vi "MVP02_P_CD.vi"() -> ()   [LabVIEW 2016]
uses:
  <vilib>/xnet/xnet.llb/XNET Read (Signal Waveform) .vi
  <vilib>/Waveform/WDTOps.llb/WDT Append Waveforms DBL.vi
  <vilib>/Waveform/WDTOps.llb/WDT Number of Waveform Samples DBL.vi
  <vilib>/measure/matone.llb/Extract Single Tone Information 1 Chan.vi
  <vilib>/measure/mamon.llb/Create Continuous Mask.vi
  <vilib>/measure/mamon.llb/Limit Testing Time.vi
  Custom Device/MVP02/MVP02 Custom Device.lvlib
  <vilib>/measure/NI_MAPro.lvlib
  <vilib>/measure/NI_MABase.lvlib
panel:
  out "error out 6":errorcluster
  out "Waveform Graph":waveform(dbl)[](graph)
  out "test passed?":bool
  out "error out 4":errorcluster
  out "error out 3":errorcluster caption="error out"
  out "error out 2":errorcluster caption="error out"
  in  "signal type":T1(ring)
  in  "error in (no error)":errorcluster
  out "error out":errorcluster
  in  "Repeticao":dbl format="%#_13g"
  in  "Caso Teste":dbl format="%#_13g"
  out "Gabarito":string
  out "String (OCR/OCV 1)":string
  out "Passed?":bool
  in  "milliseconds to wait":u32=100
  in  "stop":bool
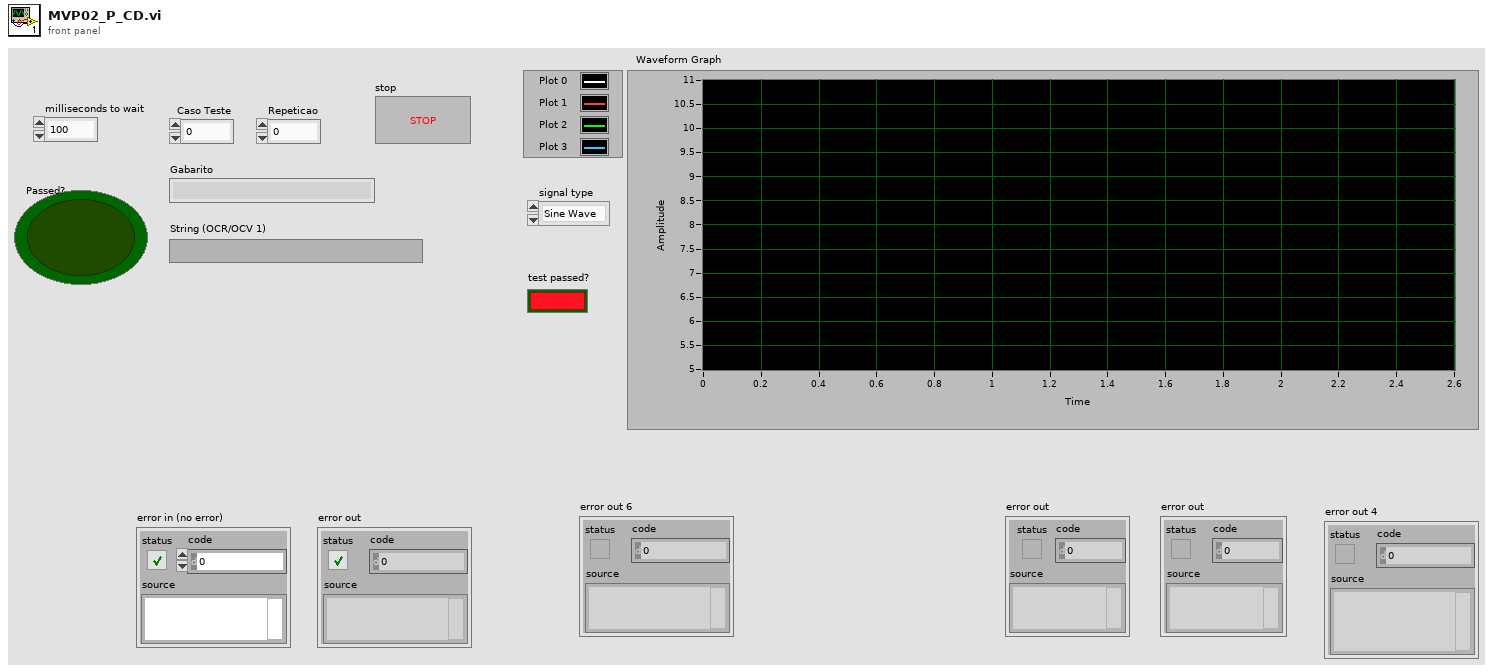
[diagram p1: front panel]
types:
  T1 = enum16{"Sine Wave", "Triangle Wave", "Square Wave", "Sawtooth Wave"}
  T2 = cluster{"pass region":i32, "include UL":bool, "include LL":bool}
  T3 = typedef "Vision Case.ctl" = enum16{"Espera", "OCR", "OCR2", "Outros"}
  T4 = typedef "IMAQ Image.ctl" = refnum<image>
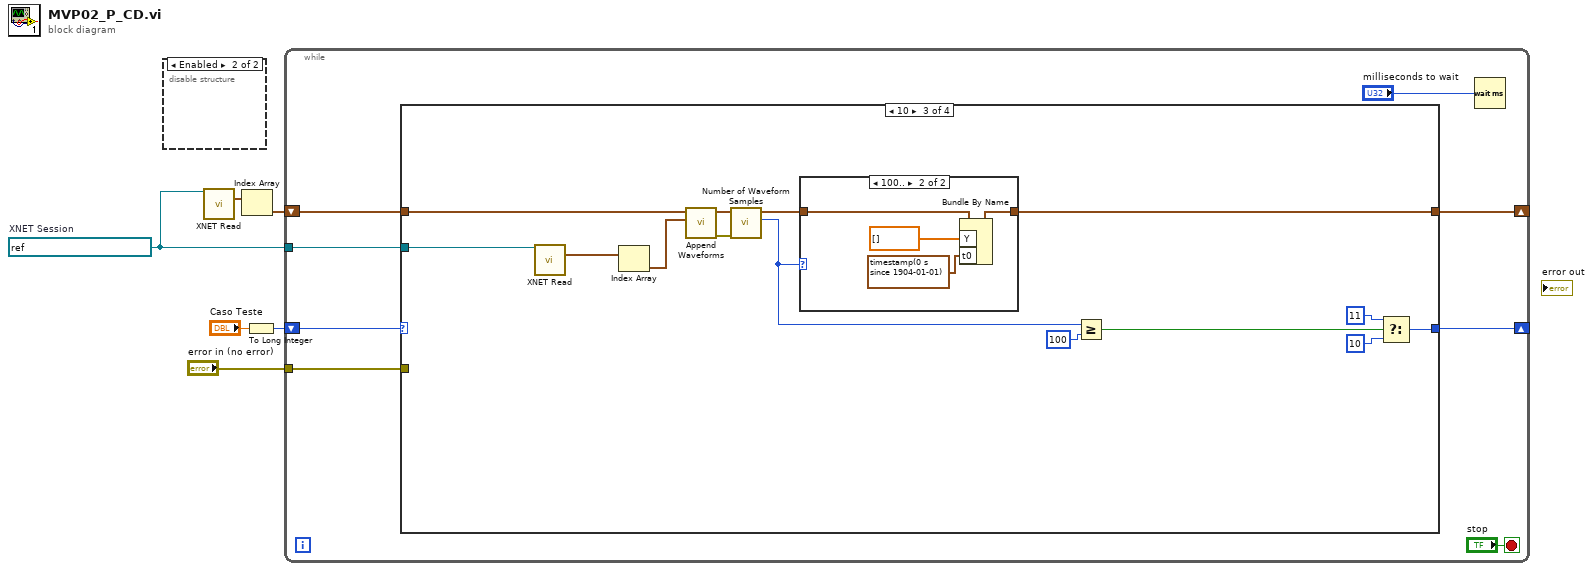
[diagram p0: block diagram]
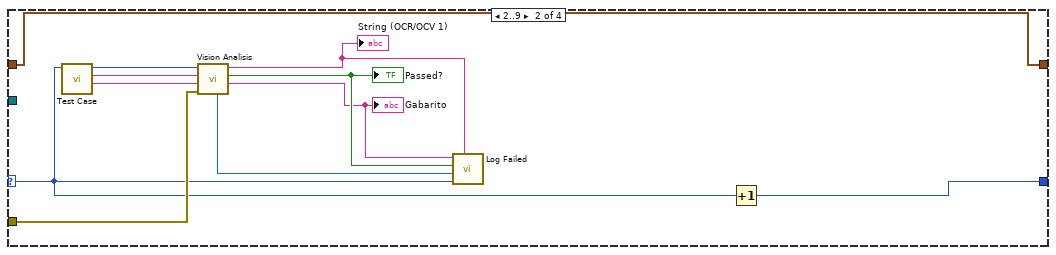
[diagram p3: hidden frame]
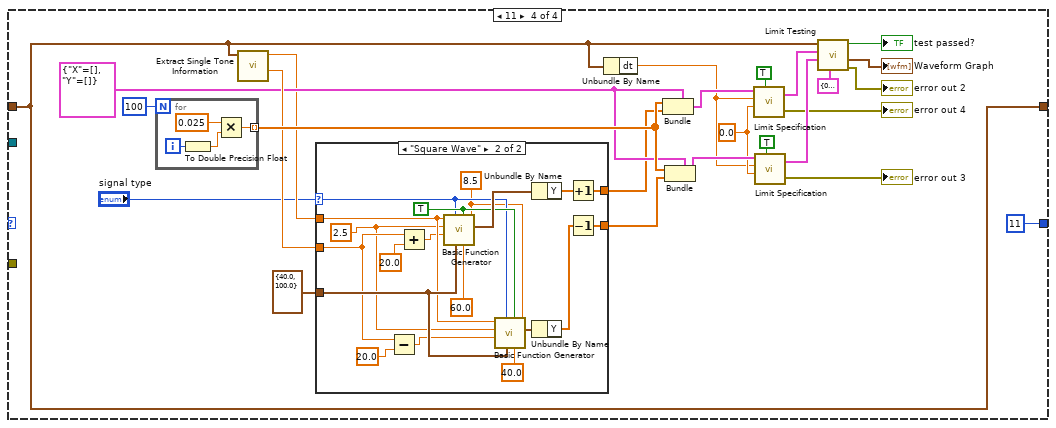
[diagram p5: hidden frame]
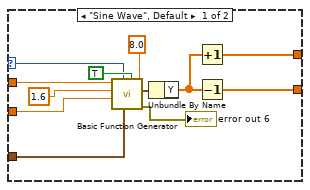
[diagram p6: hidden frame]
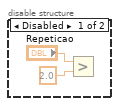
[diagram p7: hidden frame]
diagram:
  w2 = refnum<k21> "New NI-XNET Session"  # XNET Session
  n1 = disable-structure shown="Enabled" {
    frame Disabled {
      n2 = Greater?(x="Repeticao", y=2.0) -> ()  [unwired: 1 out]
    }
    frame Enabled {
    }
  }
  n3 = call-poly <vilib>:"XNET Read.vi"("session in"=w2) -> ("data"=w3:waveform(dbl)[])  [unwired: 12 in, 2 out]
  n4 = Index Array(array=w3) -> (element=w1:waveform(dbl))  [unwired: 1 in]
  n5 = To Long Integer(number="Caso Teste") -> (32bit integer=w4:i32)
  n6 = while {
    tunnel: "error in (no error)" -> [w14]
    shift-right: [w13] -> _
    shift-left: w4 -> [w12]
    tunnel: w2 -> [w11]
    shift-right: [w9] -> _
    shift-left: w1 -> [w10]
    stop <- "stop" stop-if-true
    n7 = case shown="10" w12 {
      selector: w12 -> [w18 w21 _ _]
      tunnel: w14 -> [_ w29 _ _]
      tunnel: [w18 w20 w34 11 ("32bit integer")] -> w13
      tunnel: w11 -> [_ _ w42 _]
      tunnel: w10 -> [w17 w19 w41 w50]
      tunnel: [w17 w19 w35 w50] -> w9
      frame 0, Default {
      }
      frame 2..9 {
        n8 = call "Test Case.vi"("Numeric"=w21) -> ("Linha 2"=w26:string, "Linha 1"=w27:string, "Image Case"=w28:T3)  [unwired: 8 in]
        n9 = call "Vision Analisis.vi"("error in"=w29, "Linha 2"=w26, "Linha 1"=w27, "Image Case"=w28) -> ("Gabarito"=w23:string, "Passed?"=w24:bool, "String (OCR/OCV 1)"=w22:string, "Image Out"=w25:T4)  [unwired: 3 in, 1 out]
        "Passed?" <- w24
        "String (OCR/OCV 1)" <- w22
        "Gabarito" <- w23
        n10 = call "Log Failed.vi"("RESULTADO"=w22, "Case number"=w21, "Image In"=w25, "Boolean"=w24, "GABARITO"=w23) -> ()  [unwired: 7 in]
        n11 = Increment(x=w21) -> (x+1=w20:i32)
      }
      frame 10 {
        n12 = call-poly <vilib>:"XNET Read.vi"("session in"=w42) -> ("data"=w40:waveform(dbl)[])  [unwired: 12 in, 2 out]
        n13 = Index Array(array=w40) -> (element=w39:waveform(dbl))  [unwired: 1 in]
        n14 = call-poly <vilib>:"Append Waveforms.vi"("waveform B"=w39, "waveform A"=w41) -> ("error out"=w38:errorcluster, "waveform out"=w37:waveform(dbl))  [unwired: 8 in]
        n15 = call-poly <vilib>:"Number of Waveform Samples.vi"("error in (no error)"=w38, "waveform in"=w37) -> ("number of samples"=w31:i32, "waveform out"=w36:waveform(dbl))  [unwired: 7 in, 1 out]
        n16 = case shown="100.." w31 {
          tunnel: w36 -> [w44 w45]
          tunnel: [w44 w48] -> w35
          frame 0, Default {
          }
          frame 100.. {
            n17 = Bundle By Name(cluster=w45, "Y"=dbl[] [], "t0"=timestamp(0 s since 1904-01-01)) -> (w48:waveform(dbl))
          }
        }
        n18 = Greater Or Equal?(x=w31, y=100) -> (x >= y?=w33:bool)
        n19 = Select(t=11 ("32bit integer"), s=w33, f=10 ("32bit integer")) -> (s? t:f=w34:i32)
      }
      frame 11 {
        w52 = 0.0 ("x0")
        w63 = cluster{"X":dbl[], "Y":dbl[]} {"X"=[], "Y"=[]} ("Specification Cluster")
        n20 = for {
          N: 100 -> [_]
          tunnel: [w108] -> w70 mode=indexing
          i -> [w106]
          n21 = To Double Precision Float(number=w106) -> (double precision float=w105:dbl)
          n22 = Multiply(x=0.025 ("y"), y=w105) -> (x*y=w108:dbl)
        }
        n23 = call-poly <vilib>:"Extract Single Tone Information.vi"("time signal in"=w50) -> ("detected phase (deg)"=w68:dbl, "detected frequency"=w62:dbl)  [unwired: 5 in, 4 out]
        n24 = case shown="\"Square Wave\"" "signal type" {
          selector: "signal type" -> [w80 w97]
          tunnel: cluster{"Fs":dbl, "#s":dbl} {"Fs"=40.0, "#s"=100.0} ("sampling info") -> [w85 w99]
          tunnel: w68 -> [w83 w88]
          tunnel: w62 -> [w81 w95]
          tunnel: [w78 w93] -> w60
          tunnel: [w76 w92] -> w59
          frame "Sine Wave", Default {
            n25 = call <vilib>:"Basic Function Generator.vi"("offset"=8.0, "reset signal"=TRUE, "sampling info"=w85, "signal type"=w80, "phase"=w83, "amplitude"=1.6, "frequency"=w81) -> ("error out"=→"error out 6":errorcluster, "signal out"=w79:waveform(dbl))  [unwired: 2 in, 1 out]
            n26 = Unbundle By Name(w79) -> ("Y"=w77:dbl[])
            n27 = Increment(x=w77) -> (x+1=w78:dbl[])
            n28 = Decrement(x=w77) -> (x-1=w76:dbl[])
          }
          frame "Square Wave" {
            w86 = 2.5 ("amplitude")
            w98 = TRUE ("reset signal")
            w96 = 8.5 ("offset")
            n29 = Subtract(x=w88, y=20.0) -> (x-y=w89:dbl)
            n30 = Add(x=w88, y=20.0) -> (x+y=w91:dbl)
            n31 = call <vilib>:"Basic Function Generator.vi"("offset"=w96, "square wave duty cycle (%)"=60.0 ("square wave duty cycle (%) up"), "reset signal"=w98, "sampling info"=w99, "signal type"=w97, "phase"=w91, "amplitude"=w86, "frequency"=w95) -> ("signal out"=w103:waveform(dbl))  [unwired: 1 in, 2 out]
            n32 = call <vilib>:"Basic Function Generator.vi"("offset"=w96, "square wave duty cycle (%)"=40.0 ("square wave duty cycle (%) down"), "reset signal"=w98, "sampling info"=w99, "signal type"=w97, "phase"=w89, "amplitude"=w86, "frequency"=w95) -> ("signal out"=w102:waveform(dbl))  [unwired: 1 in, 2 out]
            n33 = Unbundle By Name(w103) -> ("Y"=w101:dbl[])
            n34 = Unbundle By Name(w102) -> ("Y"=w100:dbl[])
            n35 = Increment(x=w101) -> (x+1=w93:dbl[])
            n36 = Decrement(x=w100) -> (x-1=w92:dbl[])
          }
        }
        n37 = Unbundle By Name(w50) -> ("dt"=w49:dbl)
        n38 = Bundle(cluster=w63, "X"=w70, "Y"=w60) -> (w73:cluster{"X":dbl[], "Y":dbl[]})
        n39 = Bundle(cluster=w63, "X"=w70, "Y"=w59) -> (w64:cluster{"X":dbl[], "Y":dbl[]})
        n40 = call-poly <vilib>:"Limit Specification.vi"("Specification Cluster"=w73, "dx"=w49, "x0"=w52, "Reset"=TRUE) -> ("Limit"=w67:cluster{"x0":dbl, "dx":dbl, "Y":dbl[]}, "error out"=→"error out 4":errorcluster)  [unwired: 1 in]
        n41 = call-poly <vilib>:"Limit Specification.vi"("Specification Cluster"=w64, "dx"=w49, "x0"=w52, "Reset"=TRUE) -> ("Limit"=w65:cluster{"x0":dbl, "dx":dbl, "Y":dbl[]}, "error out"=→"error out 3":errorcluster)  [unwired: 1 in]
        n42 = call-poly <vilib>:"Limit Testing.vi"("limit test config"=T2 {"pass region"=0, "include UL"=TRUE, "include LL"=TRUE}, "lower limit"=w65, "upper limit"=w67, "signal in"=w50) -> ("error out"=→"error out 2":errorcluster, "output values"=→"Waveform Graph":waveform(dbl)[], "test passed?"=→"test passed?":bool)  [unwired: 2 in, 3 out]
      }
    }
    n43 = Wait (ms)(milliseconds to wait="milliseconds to wait") -> ()  [unwired: 1 out]
  }
